vi "Módul_Idioma.vi"(8 "Idioma":string, 10 "Array":refnum<vi>[](array[refnum]), 11 "Caselles":refnum<vi>[](array[refnum])) -> (0 "TextosEstatMaquina":string[](array[string]), 2 "MissatgesUsuari":string[](array[string]))   [LabVIEW 2017]
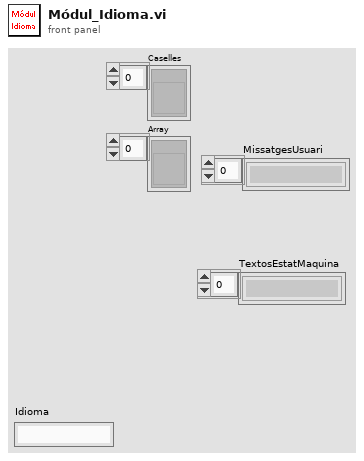
[diagram p1: front panel]
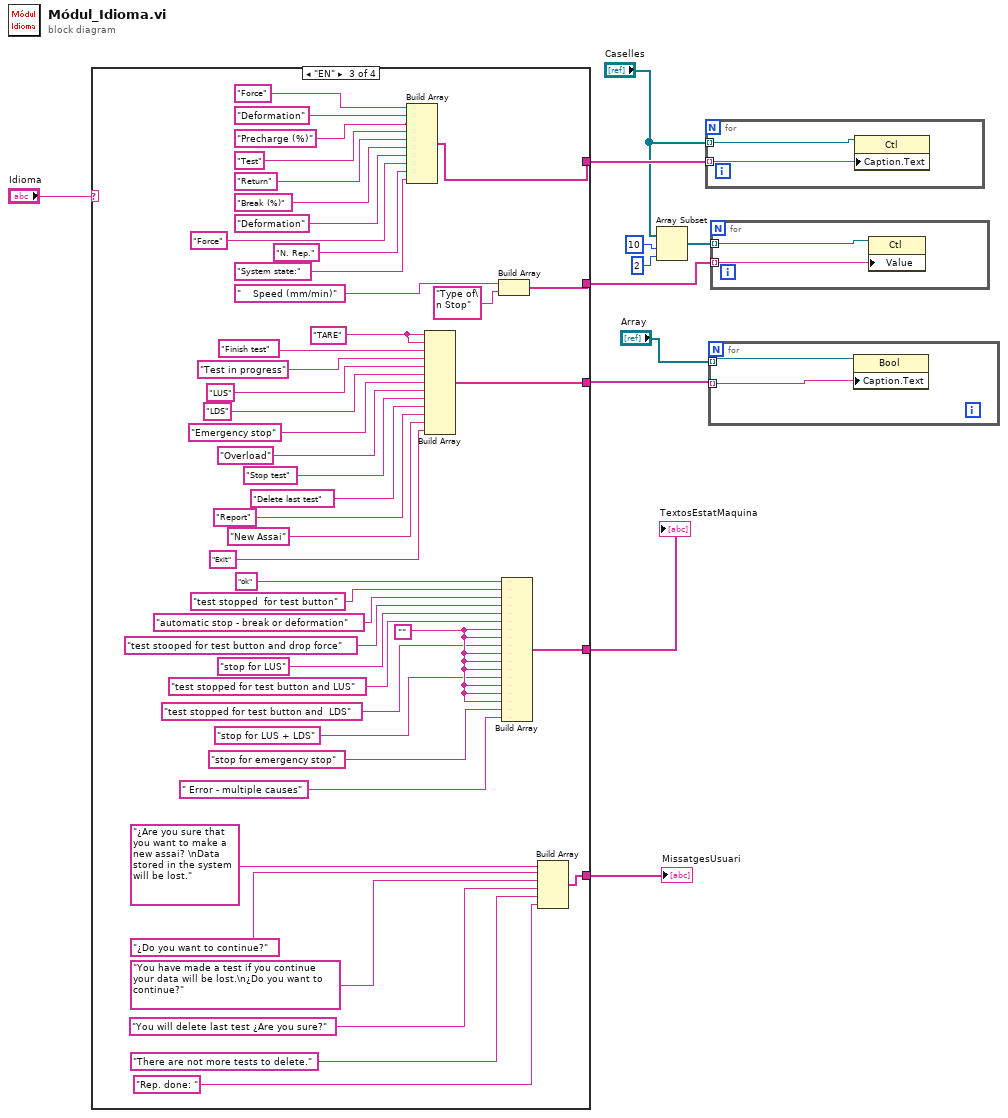
[diagram p0: block diagram]
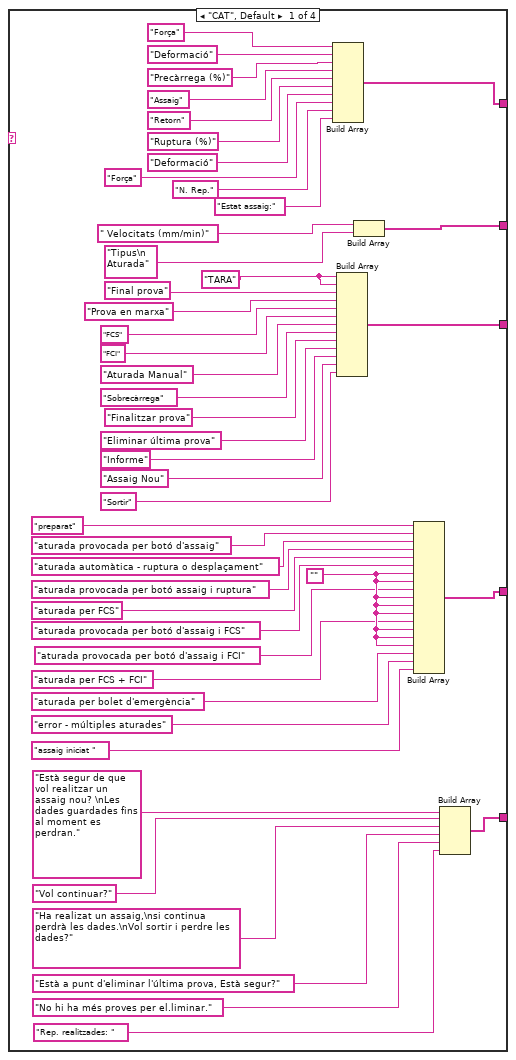
[diagram p2: hidden frame]
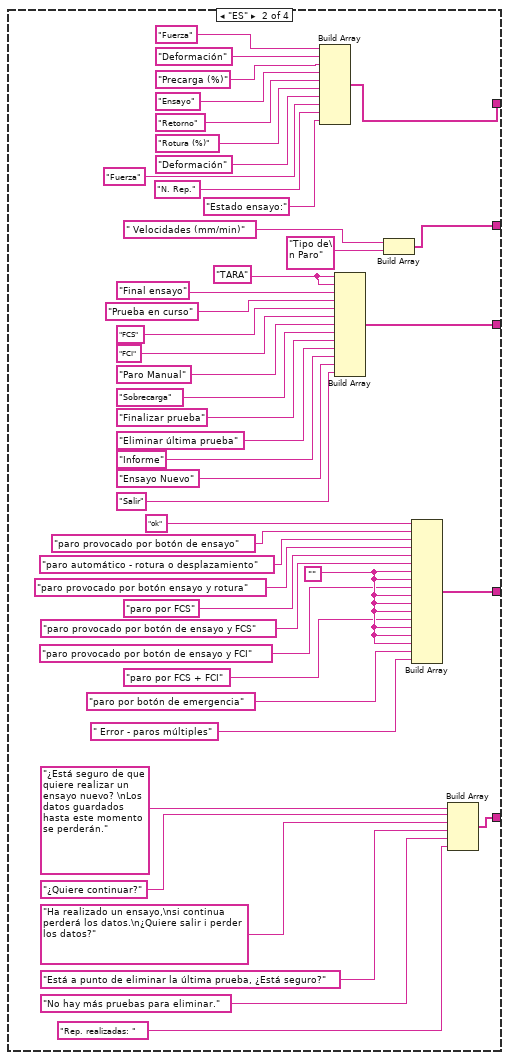
[diagram p3: hidden frame]
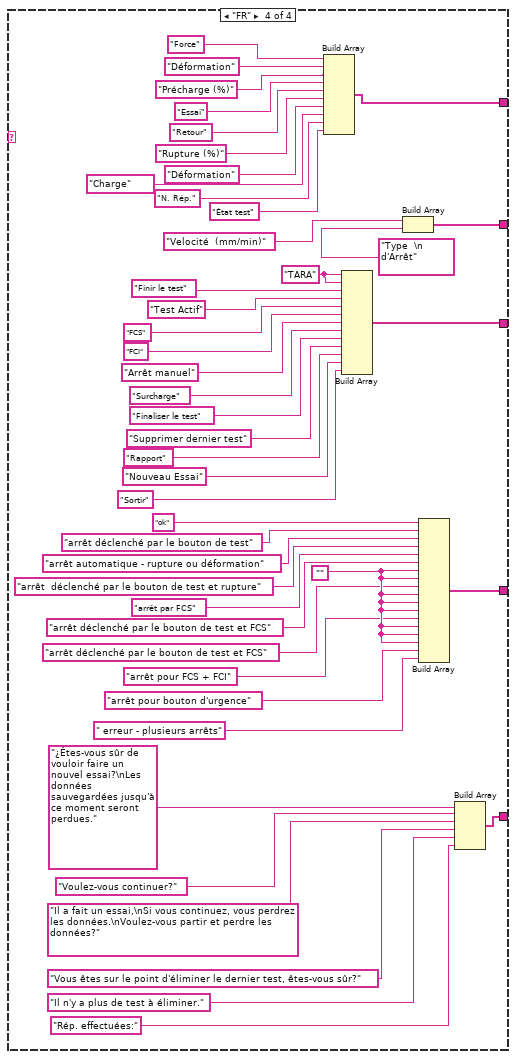
[diagram p4: hidden frame]
diagram:
  n1 = case shown="\"EN\"" "Idioma" {
    tunnel: [w27 w102 w148 w194] -> w11
    tunnel: [w26 w89 w135 w181] -> w9
    tunnel: [w25 w88 w134 w180] -> w8
    tunnel: [w22 w65 w111 w157] -> w7
    tunnel: [w15 w62 w108 w154] -> w2
    frame "CAT", Default {
      w53 = ""
      w38 = "TARA" ("Caption.Text")
      n2 = Build Array("Força" ("Caption.Text"), "Deformació" ("Caption.Text"), "Precàrrega (%)" ("Caption.Text"), "Assaig" ("Caption.Text"), "Retorn" ("Caption.Text"), "Ruptura (%)" ("Caption.Text"), "Deformació" ("Caption.Text"), "Força" ("Caption.Text"), "N. Rep." ("Caption.Text"), "Estat assaig:" ("Caption.Text")) -> (w27:string[])
      n3 = Build Array(w38, w38, "Final prova" ("Caption.Text"), "Prova en marxa" ("Caption.Text"), "FCS" ("Caption.Text"), "FCI" ("Caption.Text"), "Aturada Manual" ("Caption.Text"), "Sobrecàrrega" ("Caption.Text"), "Finalitzar prova" ("Caption.Text"), "Eliminar última prova" ("Caption.Text"), "Informe" ("Caption.Text"), "Assaig Nou" ("Caption.Text"), "Sortir" ("Caption.Text")) -> (w26:string[])
      n4 = Build Array(" Velocitats (mm/min)" ("Caption.Text"), "Tipus\n Aturada" ("Caption.Text")) -> (w15:string[])
      n5 = Build Array("preparat" ("Estado ensayo:"), "aturada provocada per botó d'assaig" ("Estado ensayo:"), "aturada automàtica - ruptura o desplaçament" ("Estado ensayo:"), "aturada provocada per botó assaig i ruptura" ("Estado ensayo:"), "aturada per FCS" ("Estado ensayo:"), "aturada provocada per botó d'assaig i FCS" ("Estado ensayo:"), w53, w53, "aturada provocada per botó d'assaig i FCI" ("Estado ensayo:"), w53, w53, w53, "aturada per FCS + FCI" ("Estado ensayo:"), w53, w53, w53, "aturada per bolet d'emergència" ("Estado ensayo:"), "error - múltiples aturades" ("Estado ensayo:"), "assaig iniciat " ("Estado ensayo:")) -> (w25:string[])
      n6 = Build Array("Està segur de que vol realitzar un assaig nou? \nLes dades guardades fins al moment es perdran.", "Vol continuar?", "Ha realizat un assaig,\nsi continua perdrà les dades.\nVol sortir i perdre les dades?", "Està a punt d'eliminar l'última prova, Està segur?", "No hi ha més proves per el.liminar.", "Rep. realitzades: ") -> (w22:string[])
    }
    frame "ES" {
      w98 = ""
      w81 = "TARA" ("Caption.Text")
      n7 = Build Array("Fuerza" ("Caption.Text"), "Deformación" ("Caption.Text"), "Precarga (%)" ("Caption.Text"), "Ensayo" ("Caption.Text"), "Retorno" ("Caption.Text"), "Rotura (%)" ("Caption.Text"), "Deformación" ("Caption.Text"), "Fuerza" ("Caption.Text"), "N. Rep." ("Caption.Text"), "Estado ensayo:" ("Caption.Text")) -> (w102:string[])
      n8 = Build Array(w81, w81, "Final ensayo" ("Caption.Text"), "Prueba en curso" ("Caption.Text"), "FCS" ("Caption.Text"), "FCI" ("Caption.Text"), "Paro Manual" ("Caption.Text"), "Sobrecarga" ("Caption.Text"), "Finalizar prueba" ("Caption.Text"), "Eliminar última prueba" ("Caption.Text"), "Informe" ("Caption.Text"), "Ensayo Nuevo" ("Caption.Text"), "Salir" ("Caption.Text")) -> (w89:string[])
      n9 = Build Array(" Velocidades (mm/min)" ("Caption.Text"), "Tipo de\n Paro" ("Caption.Text")) -> (w62:string[])
      n10 = Build Array("ok" ("Estado ensayo:"), "paro provocado por botón de ensayo" ("Estado ensayo:"), "paro automático - rotura o desplazamiento" ("Estado ensayo:"), "paro provocado por botón ensayo y rotura" ("Estado ensayo:"), "paro por FCS" ("Estado ensayo:"), "paro provocado por botón de ensayo y FCS" ("Estado ensayo:"), w98, w98, "paro provocado por botón de ensayo y FCI" ("Estado ensayo:"), w98, w98, w98, "paro por FCS + FCI" ("Estado ensayo:"), w98, w98, w98, "paro por botón de emergencia" ("Estado ensayo:"), " Error - paros múltiples" ("Estado ensayo:")) -> (w88:string[])
      n11 = Build Array("¿Está seguro de que quiere realizar un ensayo nuevo? \nLos datos guardados hasta este momento se perderán.", "¿Quiere continuar?", "Ha realizado un ensayo,\nsi continua perderá los datos.\n¿Quiere salir i perder los datos?", "Está a punto de eliminar la última prueba, ¿Está seguro?", "No hay más pruebas para eliminar.", "Rep. realizadas: ") -> (w65:string[])
    }
    frame "EN" {
      w144 = ""
      w127 = "TARE" ("Caption.Text")
      n12 = Build Array("Force" ("Caption.Text"), "Deformation" ("Caption.Text"), "Precharge (%)" ("Caption.Text"), "Test" ("Caption.Text"), "Return" ("Caption.Text"), "Break (%)" ("Caption.Text"), "Deformation" ("Caption.Text"), "Force" ("Caption.Text"), "N. Rep." ("Caption.Text"), "System state:" ("Caption.Text")) -> (w148:string[])
      n13 = Build Array(w127, w127, "Finish test" ("Caption.Text"), "Test in progress" ("Caption.Text"), "LUS" ("Caption.Text"), "LDS" ("Caption.Text"), "Emergency stop" ("Caption.Text"), "Overload" ("Caption.Text"), "Stop test" ("Caption.Text"), "Delete last test" ("Caption.Text"), "Report" ("Caption.Text"), "New Assai" ("Caption.Text"), "Exit" ("Caption.Text")) -> (w135:string[])
      n14 = Build Array("    Speed (mm/min)" ("Caption.Text"), "Type of\n Stop" ("Caption.Text")) -> (w108:string[])
      n15 = Build Array("ok" ("Estado ensayo:"), "test stopped  for test button" ("Estado ensayo:"), "automatic stop - break or deformation" ("Estado ensayo:"), "test stooped for test button and drop force" ("Estado ensayo:"), "stop for LUS" ("Estado ensayo:"), "test stopped for test button and LUS" ("Estado ensayo:"), w144, w144, "test stopped for test button and  LDS" ("Estado ensayo:"), w144, w144, w144, "stop for LUS + LDS" ("Estado ensayo:"), w144, w144, w144, "stop for emergency stop" ("Estado ensayo:"), " Error - multiple causes" ("Estado ensayo:")) -> (w134:string[])
      n16 = Build Array("¿Are you sure that you want to make a new assai? \nData stored in the system will be lost.", "¿Do you want to continue?", "You have made a test if you continue your data will be lost.\n¿Do you want to continue?", "You will delete last test ¿Are you sure?", "There are not more tests to delete.", "Rep. done: ") -> (w111:string[])
    }
    frame "FR" {
      w190 = ""
      w173 = "TARA" ("Caption.Text")
      n17 = Build Array("Force" ("Caption.Text"), "Déformation" ("Caption.Text"), "Précharge (%)" ("Caption.Text"), "Essai" ("Caption.Text"), "Retour" ("Caption.Text"), "Rupture (%)" ("Caption.Text"), "Déformation" ("Caption.Text"), "Charge" ("Caption.Text"), "N. Rép." ("Caption.Text"), "État test" ("Caption.Text")) -> (w194:string[])
      n18 = Build Array(w173, w173, "Finir le test" ("Caption.Text"), "Test Actif" ("Caption.Text"), "FCS" ("Caption.Text"), "FCI" ("Caption.Text"), "Arrêt manuel" ("Caption.Text"), "Surcharge" ("Caption.Text"), "Finaliser le test" ("Caption.Text"), "Supprimer dernier test" ("Caption.Text"), "Rapport" ("Caption.Text"), "Nouveau Essai" ("Caption.Text"), "Sortir" ("Caption.Text")) -> (w181:string[])
      n19 = Build Array("Velocité  (mm/min)" ("Caption.Text"), "Type  \n d'Arrêt" ("Caption.Text")) -> (w154:string[])
      n20 = Build Array("ok" ("Estado ensayo:"), "arrêt déclenché par le bouton de test" ("Estado ensayo:"), "arrêt automatique - rupture ou déformation" ("Estado ensayo:"), "arrêt  déclenché par le bouton de test et rupture" ("Estado ensayo:"), "arrêt par FCS" ("Estado ensayo:"), "arrêt déclenché par le bouton de test et FCS" ("Estado ensayo:"), w190, w190, "arrêt déclenché par le bouton de test et FCS" ("Estado ensayo:"), w190, w190, w190, "arrêt pour FCS + FCI" ("Estado ensayo:"), w190, w190, w190, "arrêt pour bouton d'urgence" ("Estado ensayo:"), " erreur - plusieurs arrêts" ("Estado ensayo:")) -> (w180:string[])
      n21 = Build Array("¿Êtes-vous sûr de vouloir faire un nouvel essai?\nLes données sauvegardées jusqu'à ce moment seront perdues.", "Voulez-vous continuer?", "Il a fait un essai,\nSi vous continuez, vous perdrez les données.\nVoulez-vous partir et perdre les données?", "Vous êtes sur le point d'éliminer le dernier test, êtes-vous sûr?", "Il n'y a plus de test à éliminer.", "Rép. effectuées:") -> (w157:string[])
    }
  }
  "TextosEstatMaquina" <- w8
  "MissatgesUsuari" <- w7
  n22 = Array Subset(array="Caselles", index=10, length=2) -> (w3:refnum<vi>[])
  n23 = for {
    tunnel: w11 -> [w198] mode=indexing
    tunnel: "Caselles" -> [w197] mode=indexing
    n24 = property class="Ctl"(reference=w197, "Caption.Text"=w198) -> ()  [unwired: 1 in, 2 out]
  }
  n25 = for {
    tunnel: "Array" -> [w200] mode=indexing
    tunnel: w9 -> [w199] mode=indexing
    n26 = property class="Bool"(reference=w200, "Caption.Text"=w199) -> ()  [unwired: 1 in, 2 out]
  }
  n27 = for {
    tunnel: w2 -> [w202] mode=indexing
    tunnel: w3 -> [w201] mode=indexing
    n28 = property class="Ctl"(reference=w201, "Value"=w202) -> ()  [unwired: 1 in, 2 out]
  }
